vi "ReentrantDriver.vi"() -> ()   [LabVIEW 2012]
panel:
  out "NumOut 2":dbl
  out "NumOut":dbl
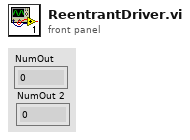
[diagram p1: front panel]
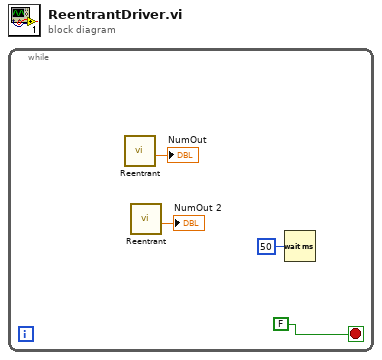
[diagram p0: block diagram]
diagram:
  n1 = while {
    stop <- FALSE stop-if-true
    n2 = call "Reentrant.vi"() -> ("NumOut"=→"NumOut":dbl)  [unwired: 11 in]
    n3 = call "Reentrant.vi"() -> ("NumOut"=→"NumOut 2":dbl)  [unwired: 11 in]
    n4 = Wait (ms)(milliseconds to wait=u32 50) -> ()  [unwired: 1 out]
  }
